vi "Database Template path.vi"() -> (3 "Access path":path)   [LabVIEW 2019]
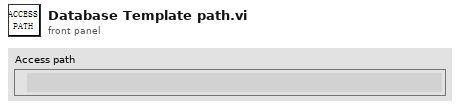
[diagram p1: front panel]
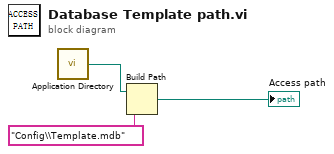
[diagram p0: block diagram]
diagram:
  n1 = call <vilib>:"Application Directory.vi"() -> ("Application Directory"=w3:path)
  n2 = Build Path(base path=w3, name or relative path="Config\\Template.mdb" ("名称或相对路径")) -> (appended path=→"Access path":path)
